vi "Export to CSV.vi"(8 "error in":errorcluster, 10 "VI Information Array":T1[](array[typedef]), 11 "Engine in":refnum<class "Engine.lvclass">) -> (0 "error out":errorcluster, 3 "Engine out":refnum<class "Engine.lvclass">)   [LabVIEW 2019, in "Engine.lvclass"]
uses:
  Engine.lvclass
  VI Information.ctl
  <vilib>/Utility/file.llb/Write Delimited Spreadsheet (string).vi
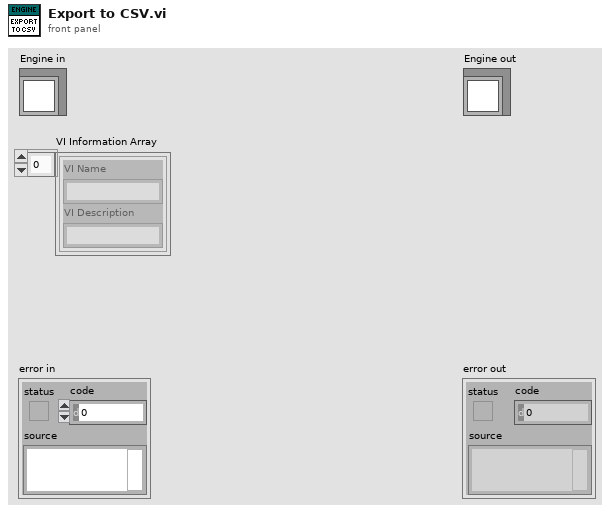
[diagram p1: front panel]
types:
  T1 = typedef "Engine.lvclass/VI Information.ctl" = cluster{"VI Name":string, "VI Description":string}
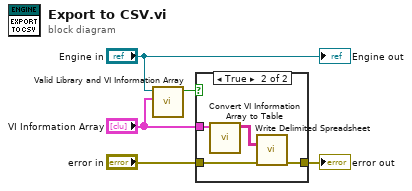
[diagram p0: block diagram]
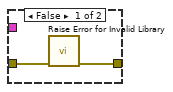
[diagram p2: hidden frame]
diagram:
  n1 = call "Valid Library and VI Information Array.vi"("VI Information Array"="VI Information Array", "Engine in"="Engine in") -> ("Valid"=w2:bool)  [unwired: 9 in]
  n2 = case shown="True" w2 {
    tunnel: [w6 w11] -> w5
    tunnel: "error in" -> [w7 w10]
    tunnel: "VI Information Array" -> [_ w9]
    frame False {
      n3 = call "Raise Error for Invalid Library.vi"("error in"=w7) -> ("error out"=w6:errorcluster)  [unwired: 10 in]
    }
    frame True {
      n4 = call "Convert VI Information Array to Table.vi"("VI Information Array"=w9) -> ("Array Out"=w8:string[][])  [unwired: 10 in]
      n5 = call-poly <vilib>:"Write Delimited Spreadsheet.vi"("2D data"=w8, "error in (no error)"=w10) -> ("error out"=w11:errorcluster)  [unwired: 12 in, 1 out]
    }
  }
  "error out" <- w5
  "Engine out" <- "Engine in"
